vi "Compare Target and Start in PowerDown.vi"(0 "Target Value":dbl[](array[numeric])=[2.0, 0.0, -5.0, -3.0, 0.0], 5 "Start Value":dbl[](array[numeric])=[5.0, 2.0, 5.0, -5.0, -5.0]) -> (4 "Valid ?":bool[](array[boolean]))   [LabVIEW 2024, in "devicePowerSequencerCoreLogic.lvlib"]
uses:
  devicePowerSequencerCoreLogic.lvlib
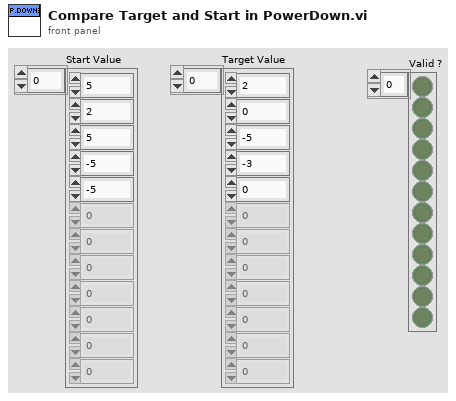
[diagram p1: front panel]
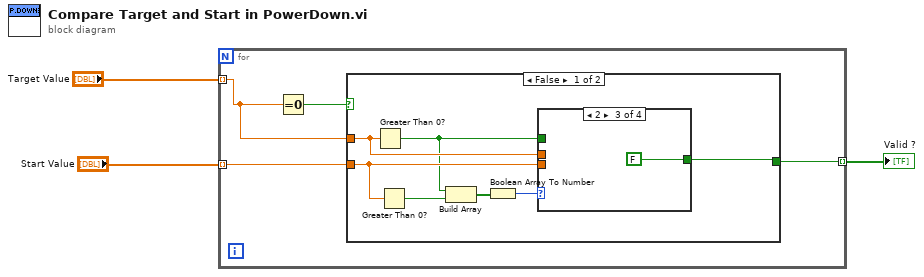
[diagram p0: block diagram]
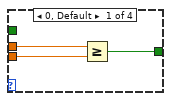
[diagram p2: hidden frame]
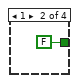
[diagram p3: hidden frame]
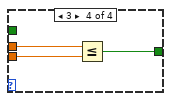
[diagram p4: hidden frame]
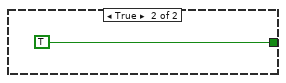
[diagram p5: hidden frame]
diagram:
  n1 = for {
    tunnel: "Target Value" -> [w5] mode=indexing
    tunnel: "Start Value" -> [w6] mode=indexing
    tunnel: [w4] -> w1 mode=indexing
    n2 = Equal To 0?(x=w5) -> (x = 0?=w7:bool)
    n3 = case shown="False" w7 {
      tunnel: w6 -> [w12 _]
      tunnel: w5 -> [w14 _]
      tunnel: [w13 TRUE] -> w4
      frame False {
        n4 = Greater Than 0?(x=w14) -> (x > 0?=w10:bool)
        n5 = Greater Than 0?(x=w12) -> (x > 0?=w11:bool)
        n6 = Build Array(w10, w11) -> (w9:bool[])
        n7 = Boolean Array To Number(Boolean array=w9) -> (number=w8:u32)
        n8 = case shown="2" w8 {
          tunnel: w12 -> [w17 _ _ w22]
          tunnel: w14 -> [w16 _ _ w20]
          tunnel: [w15 FALSE FALSE w21] -> w13
          tunnel: w10 -> [_ _ _ _]
          frame 0, Default {
            n9 = Greater Or Equal?(x=w16, y=w17) -> (x >= y?=w15:bool)
          }
          frame 1 {
          }
          frame 2 {
          }
          frame 3 {
            n10 = Less Or Equal?(x=w20, y=w22) -> (x <= y?=w21:bool)
          }
        }
      }
      frame True {
      }
    }
  }
  "Valid ?" <- w1
